vi "Game Controller scale.vi"(2 "Game controller in":i32) -> (0 "Arm out":u32)   [LabVIEW 2015]
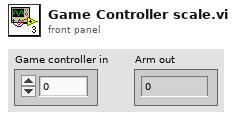
[diagram p1: front panel]
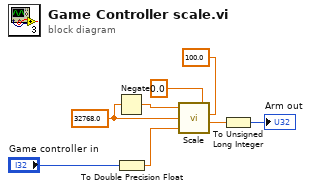
[diagram p0: block diagram]
diagram:
  w5 = 32768.0 ("Max in")
  n1 = Negate(x=w5) -> (-x=w4:dbl)
  n2 = To Double Precision Float(number="Game controller in") -> (double precision float=w6:dbl)
  n3 = call "Scale.vi"("From Min"=w4, "From Max"=w5, "Input Val"=w6, "To Min"=0.0, "To Max"=100.0) -> ("Output val"=w3:dbl)  [unwired: 1 out]
  n4 = To Unsigned Long Integer(number=w3) -> (unsigned 32bit integer=→"Arm out":u32)
